vi "Disabled.vi"(7 "Robot Mode":T2=enum."Teleop Disabled", 10 "Match Info":T1={"Autonomous Elapsed Seconds"=0.0, "TeleOp Elapsed Seconds"=0.0, "Disabled Elapsed Seconds"=93.761, "Visited Autonomous"=FALSE, "Visited TeleOp"=FALSE, "Visited Disabled"=TRUE, "Autonomous Settings"={"Autonomous Style"=enum."Independent", "VI Refnum"=refnum}}, 11 "Call Context":T3=enum."Execute") -> ()   [LabVIEW 2015]
doc: "This VI is called each time a disabled packet is received from the DS. It is often used to prepare for the next robot mode, to calibrate sensors, etc."
uses:
  <vilib>/Rock Robotics/WPI/DriverStation/WPI_DriverStationDerivedRobotMode.ctl
  <vilib>/Rock Robotics/WPI/DriverStation/WPI_DriverStationRobotMode2.ctl
  <vilib>/Rock Robotics/WPI/DriverStation/WPI_DriverStationMatch Info.ctl
  SonarAction.ctl
  Example_Code/PressureSensor/PressureSensorAction.ctl
  SingleSolenoidAction.ctl
  RefnameEnum.ctl
  TankDriveAction.ctl
panel:
  out "KinectHot?":bool
  in  "AutoID":i32=3061
  out "LCDTimer":u32=121
  out "LCDIterations":i32
  out "error out":errorcluster
  in  "error in":errorcluster
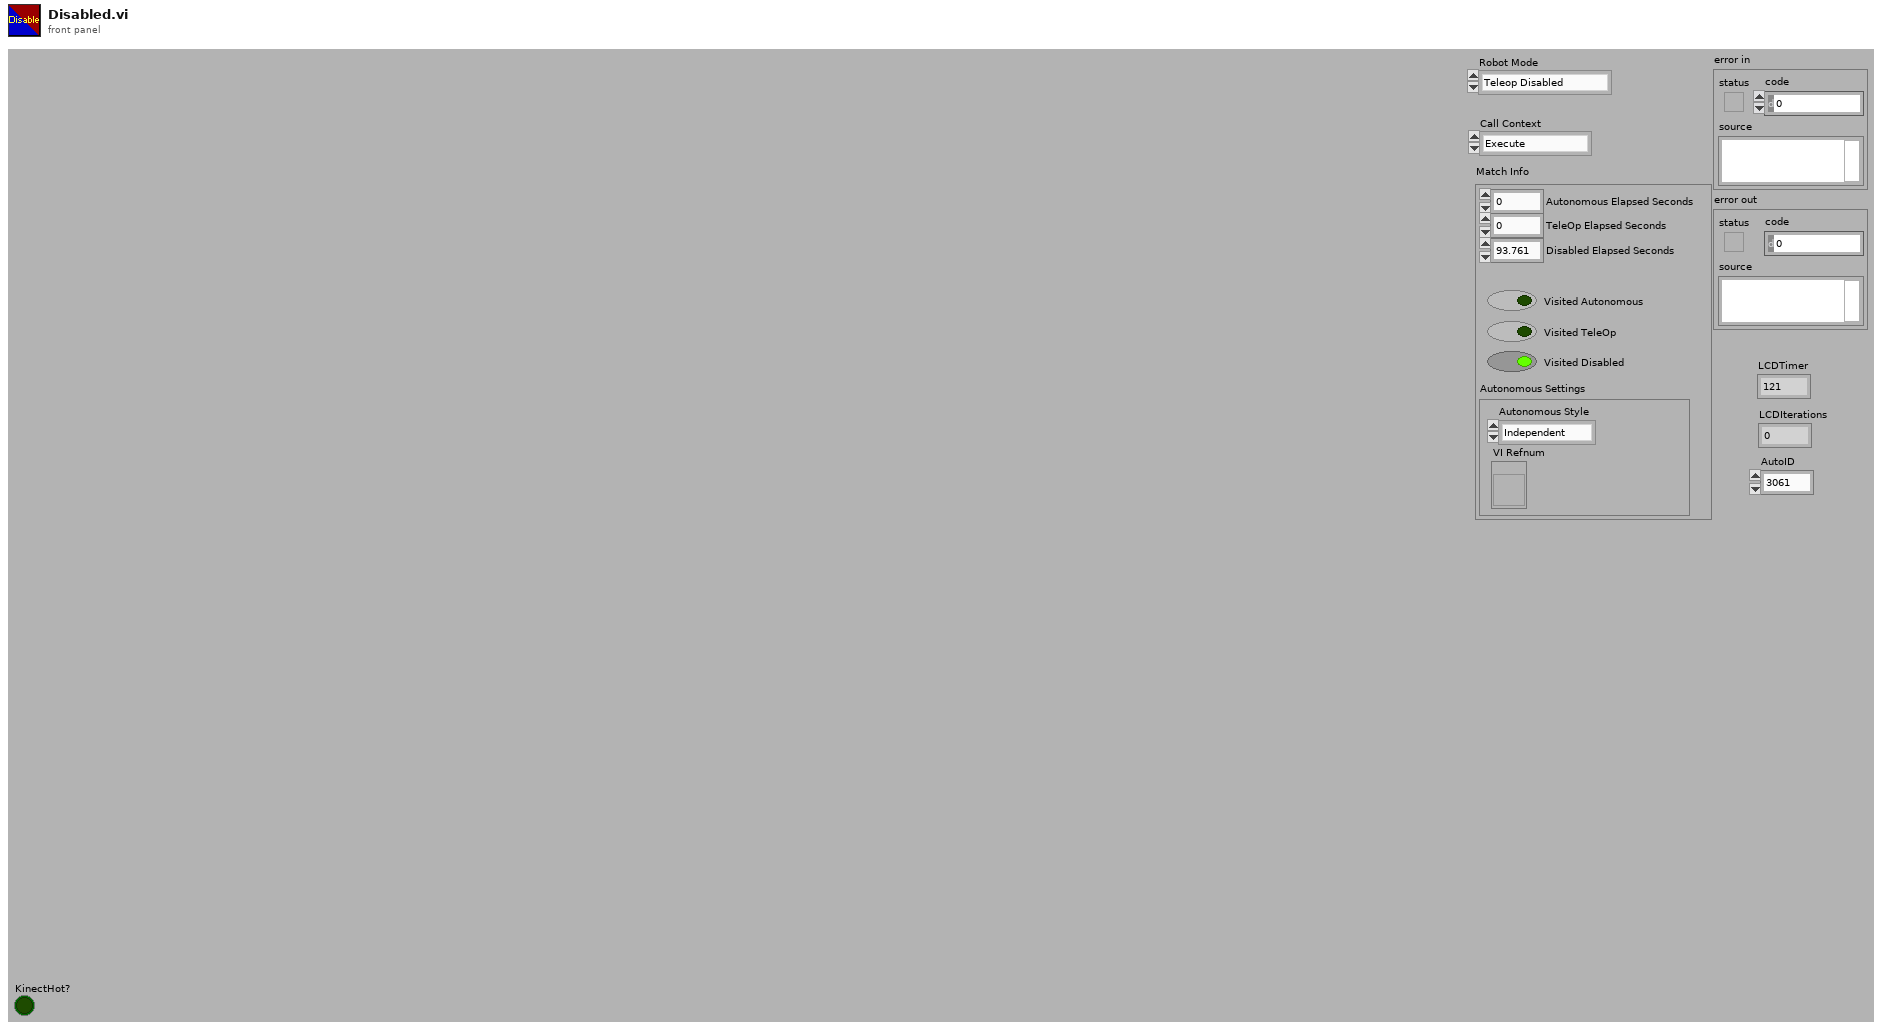
[diagram p1: front panel]
types:
  T1 = typedef "WPI_DriverStationMatch Info.ctl" = cluster{"Autonomous Elapsed Seconds":dbl, "TeleOp Elapsed Seconds":dbl, "Disabled Elapsed Seconds":dbl, "Visited Autonomous":bool, "Visited TeleOp":bool, "Visited Disabled":bool, "Autonomous Settings":cluster{"Autonomous Style":enum16{"Iterative", "Independent"}, "VI Refnum":refnum<vi>}}
  T2 = typedef "WPI_DriverStationRobotMode2.ctl" = enum16{"Autonomous Disabled", "Autonomous Enabled", "Teleop Disabled", "Teleop Enabled", "Disconnected", "Finish", "Test Disabled", "Test Enabled"}
  T3 = typedef "WPI_DriverStationDerivedRobotMode.ctl" = enum16{"Init", "Execute", "Stop"}
  T4 = typedef "TankDriveAction.ctl" = enum16{"Init", "LinearDrive", "SetValue", "Disable"}
  T5 = typedef "RefnameEnum.ctl" = enum16{"TankDrive", "Controller1", "Controller2", "SonicShifter", "Compressor"}
  T6 = typedef "SingleSolenoidAction.ctl" = enum16{"Init", "SetState", "Disable"}
  T7 = typedef "WPI_SolenoidDevRef.ctl" = cluster{"DevStatus":errorcluster, "Solenoid Module":T8, "Forward Solenoid Channel":T9, "Reverse Solenoid Channel":T9}
  T8 = typedef "FPGA_TypedefSolenoidModule.ctl" = enum16{"Solenoid Module 1", "Solenoid Module 2"}
  T9 = typedef "WPI_SolenoidChannel.ctl" = enum8{"Solenoid 1", "Solenoid 2", "Solenoid 3", "Solenoid 4", "Solenoid 5", "Solenoid 6", "Solenoid 7", "Solenoid 8", "Invalid"}
  T10 = typedef "PressureSensorAction.ctl" = enum16{"Init", "ReadValue", "Disable"}
  T11 = typedef "SonarAction.ctl" = enum16{"Init", "ReadValue", "Disable"}
  T12 = typedef "AutoMode.ctl" = enum16{"OneBallFront", "OneBallCollector", "TwoBallNormal", "TwoBallHot"}
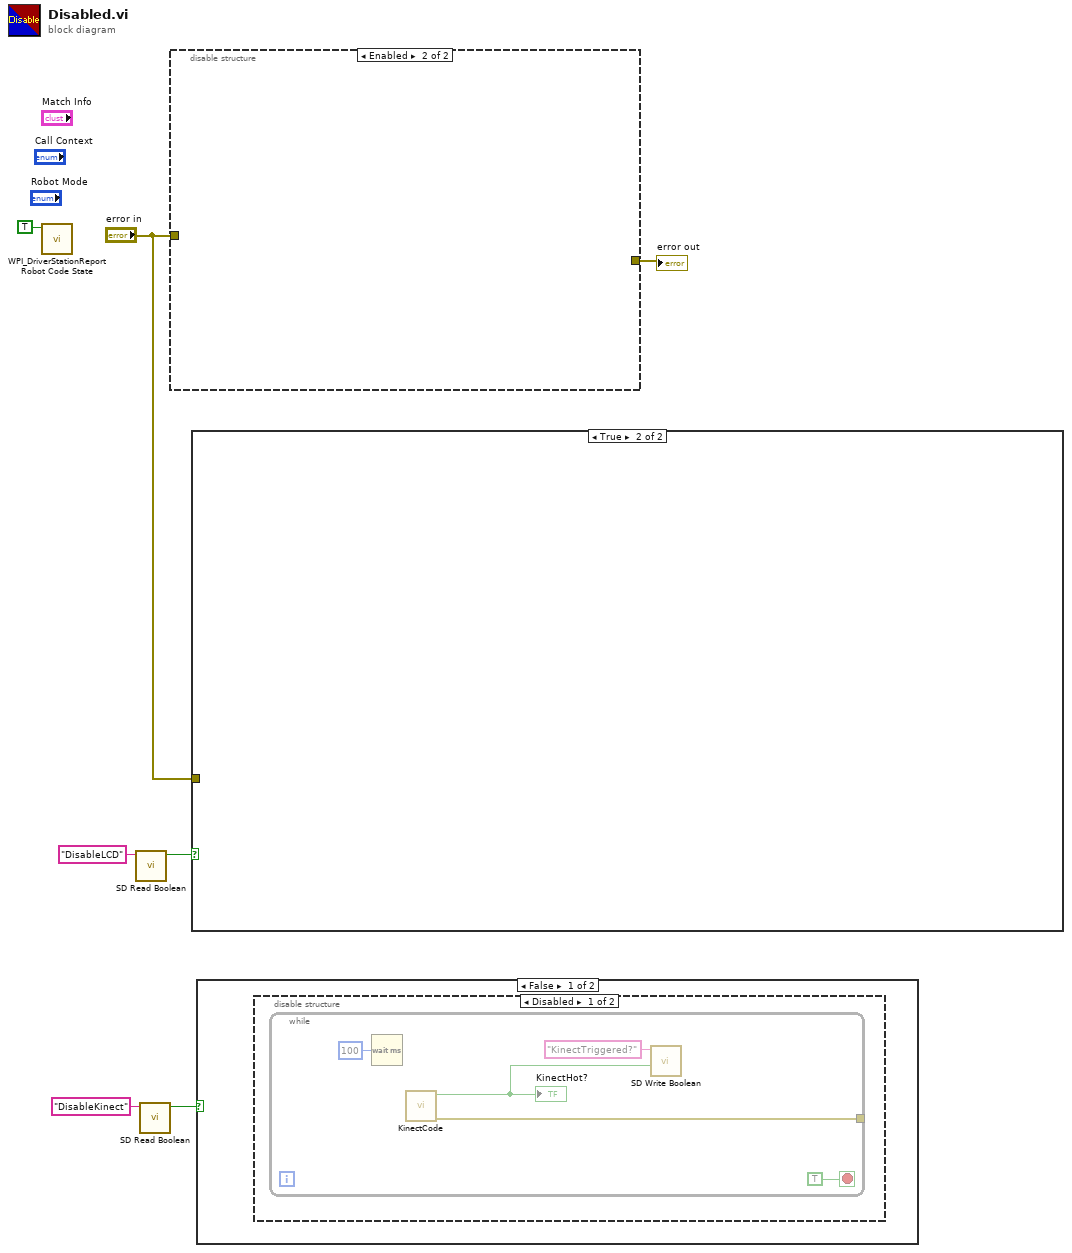
[diagram p0: block diagram]
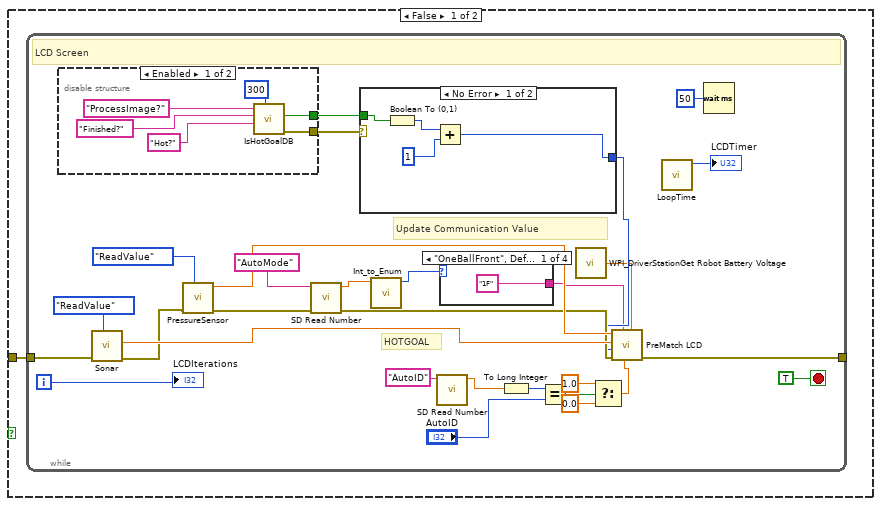
[diagram p4: hidden frame]
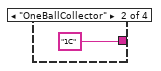
[diagram p6: hidden frame]
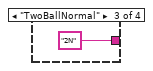
[diagram p7: hidden frame]
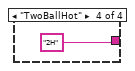
[diagram p8: hidden frame]
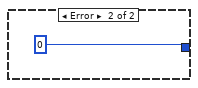
[diagram p9: hidden frame]
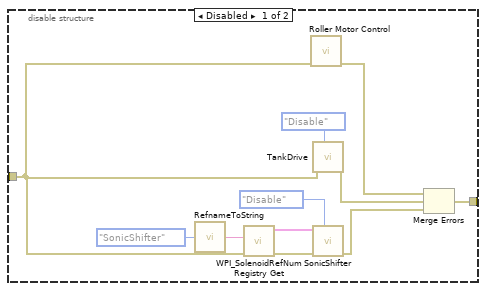
[diagram p10: hidden frame]
diagram:
  n1 = call <vilib>:"WPI_DriverStationReport Robot Code State.vi"("Disabled"=TRUE ("Autonomous")) -> ()  [unwired: 10 in, 1 out]
  n2 = call <vilib>:"SD Read Boolean.vi"("Name"="DisableLCD") -> ("Boolean"=w4:bool)  [unwired: 8 in, 2 out]
  n3 = call <vilib>:"SD Read Boolean.vi"("Name"="DisableKinect") -> ("Boolean"=w1:bool)  [unwired: 8 in, 2 out]
  n4 = disable-structure shown="Enabled" {
    disable-tunnel: [w11 _] -> w6
    disable-tunnel: "error in" -> [w10 _]
    frame Disabled {
      n5 = call "RefnameToString.vi"("Enum"=RefnameEnum."SonicShifter") -> ("Refname"=w16:string)
      n6 = call <vilib>:"WPI_SolenoidRefNum Registry Get.vi"("error in (no error)"=w10, "refnum name"=w16) -> ("error out"=w14:errorcluster, "SolenoidDevRef"=w18:T7)  [unwired: 8 in]
      n7 = call "Roller Motor Control.vi"("Error in"=w10) -> ("Error out"=w9:errorcluster)  [unwired: 10 in]
      n8 = call "TankDrive.vi"("DriveAction"=TankDriveAction."Disable", "error in (no error)"=w10) -> ("error out"=w13:errorcluster)  [unwired: 8 in, 1 out]
      n9 = call "SonicShifter.vi"("Action"=SingleSolenoidAction."Disable" ("Mode"), "error in (no error)"=w14, "SolenoidDevRef"=w18) -> ("error out"=w12:errorcluster)  [unwired: 8 in]
      n10 = Merge Errors(w9, w13, w12) -> (w11:errorcluster)
    }
    frame Enabled {
    }
  }
  "error out" <- w6
  n11 = case shown="True" w4 {
    tunnel: "error in" -> [w19 _]
    frame False {
      n12 = while {
        tunnel: w19 -> [w46]
        tunnel: [w47] -> _
        i -> [w28]
        stop <- TRUE stop-if-true
        # "HOTGOAL"
        # "Update Communication Value"
        # "LCD Screen"
        n13 = disable-structure shown="Enabled" {
          disable-tunnel: [w54 _] -> w37
          disable-tunnel: [w53 _] -> w36
          frame Enabled {
            n14 = call "IsHotGoalDB.vi"("Timeout (ms)"=u32 300, "DBHot?"="Hot?", "DBFinished?"="Finished?", "DBStart"="ProcessImage?") -> ("error out"=w54:errorcluster, "Hot?"=w53:bool)  [unwired: 4 in, 2 out]
          }
          frame Disabled {
          }
        }
        n15 = call "Sonar.vi"("Action"=SonarAction."ReadValue", "error in (no error)"=w46) -> ("error out"=w43:errorcluster, "distance"=w45:dbl)  [unwired: 8 in]
        n16 = call "PressureSensor.vi"("Action"=PressureSensorAction."ReadValue", "error in (no error)"=w43) -> ("error out"=w40:errorcluster, "Pressure"=w42:dbl)  [unwired: 8 in]
        n17 = call <vilib>:"SD Read Number.vi"("error in"=w40, "Name"="AutoMode") -> ("error out"=w39:errorcluster, "Numeric"=w33:dbl)  [unwired: 7 in, 1 out]
        n18 = case shown="No Error" w37 {
          tunnel: w36 -> [w62 _]
          tunnel: [w59 0] -> w35
          frame No Error {
            n19 = Boolean To (0,1)(Boolean=w62) -> (0, 1=w61:i16)
            n20 = Add(x=w61, y=1) -> (x+y=w59:i32)
          }
          frame Error {
          }
        }
        n21 = call "Int_to_Enum.vi"("IntIn"=w33) -> ("EnumOut"=w32:T12)  [unwired: 10 in]
        n22 = call <vilib>:"SD Read Number.vi"("Name"="AutoID") -> ("Numeric"=w26:dbl)  [unwired: 8 in, 2 out]
        n23 = case shown="\"OneBallFront\", Default" w32 {
          tunnel: ["1F" "1C" "2N" "2H"] -> w31
          frame "OneBallFront", Default {
          }
          frame "OneBallCollector" {
          }
          frame "TwoBallNormal" {
          }
          frame "TwoBallHot" {
          }
        }
        n24 = To Long Integer(number=w26) -> (32bit integer=w25:i32)
        n25 = Equal?(x=w25, y="AutoID") -> (x = y?=w23:bool)
        n26 = call <vilib>:"WPI_DriverStationGet Robot Battery Voltage.vi"() -> ("robot battery voltage"=w34:dbl)  [unwired: 14 in, 1 out]
        n27 = Select(t=1.0, s=w23, f=0.0) -> (s? t:f=w20:dbl)
        n28 = call "PreMatch LCD.vi"("Battery Voltage"=w34, "Communication Value:"=w20, "Autonomous Mode"=w31, "error in"=w39, "Camera"=w35, "Distance"=w45, "PSI"=w42) -> ("error out"=w47:errorcluster)  [unwired: 4 in]
        n29 = call "LoopTime.vi"() -> ("LoopTime"=→"LCDTimer":u32)  [unwired: 11 in]
        n30 = Wait (ms)(milliseconds to wait=u32 50) -> ()  [unwired: 1 out]
        "LCDIterations" <- w28
      }
    }
    frame True {
    }
  }
  n31 = case shown="False" w1 {
    frame False {
      n32 = disable-structure shown="Disabled" {
        frame Disabled {
          n33 = while {
            tunnel: [w66] -> _
            stop <- TRUE stop-if-true
            n34 = Wait (ms)(milliseconds to wait=u32 100) -> ()  [unwired: 1 out]
            n35 = call "KinectCode.vi"() -> ("error out"=w66:errorcluster, "HandsApart?"=w65:bool)  [unwired: 10 in]
            "KinectHot?" <- w65
            n36 = call <vilib>:"SD Write Boolean.vi"("Boolean"=w65, "Name"="KinectTriggered?") -> ()  [unwired: 8 in, 2 out]
          }
        }
        frame Enabled {
        }
      }
    }
    frame True {
    }
  }
